vi "Time Variable.vi"() -> ()   [LabVIEW 2010]
panel:
  in  "Time in Sec":dbl
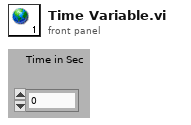
[diagram p1: front panel]
diagram:
